vi "Q.Send Function Command and wait on Ret Data.vi"(5 "Timeout(ms)":i32=100, 7 "Q Name":string, 8 "error in":errorcluster, 9 "Data1":variant, 10 "Cmd":string, 11 "Q In":refnum<queue>) -> (0 "error out":errorcluster, 2 "Ret":variant)   [LabVIEW 2024, in "EQMF.lvlib" / "Queue Utils.lvlib"]
uses:
  Queue Utils.lvlib
  Q.Element.ctl
  Q.Msg Return Info.ctl
  Q.Msg Return Data Container.ctl
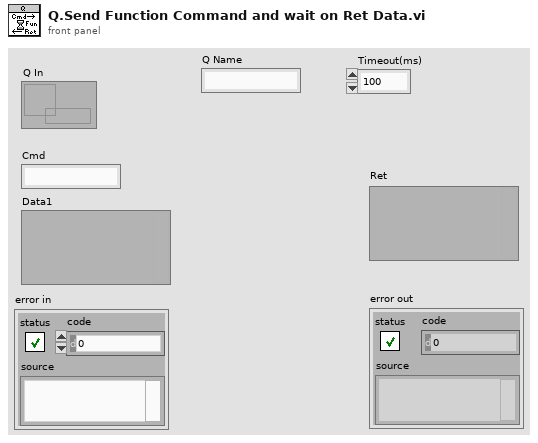
[diagram p1: front panel]
types:
  T1 = typedef "EQMF.lvlib/Queue Utils.lvlib/Q.Msg Return Info.ctl" = cluster{"Ret Q":refnum<queue>, "Ret Msg":T2, "SeqNum":i32}
  T2 = typedef "EQMF.lvlib/Queue Utils.lvlib/Q.Element.ctl" = cluster{"Cmd":string, "Sub":string, "Data1":variant, "Data2":variant}
  T3 = typedef "EQMF.lvlib/Queue Utils.lvlib/Q.Msg Return Data Container.ctl" = cluster{"SeqNum":i32, "Data":variant, "Error":errorcluster}
  T4 = cluster{"Q Cmd":refnum<queue>, "Q Ret":refnum<queue>, "Q Name":string, "Cmd ":string, "State":string, "Ret":variant}
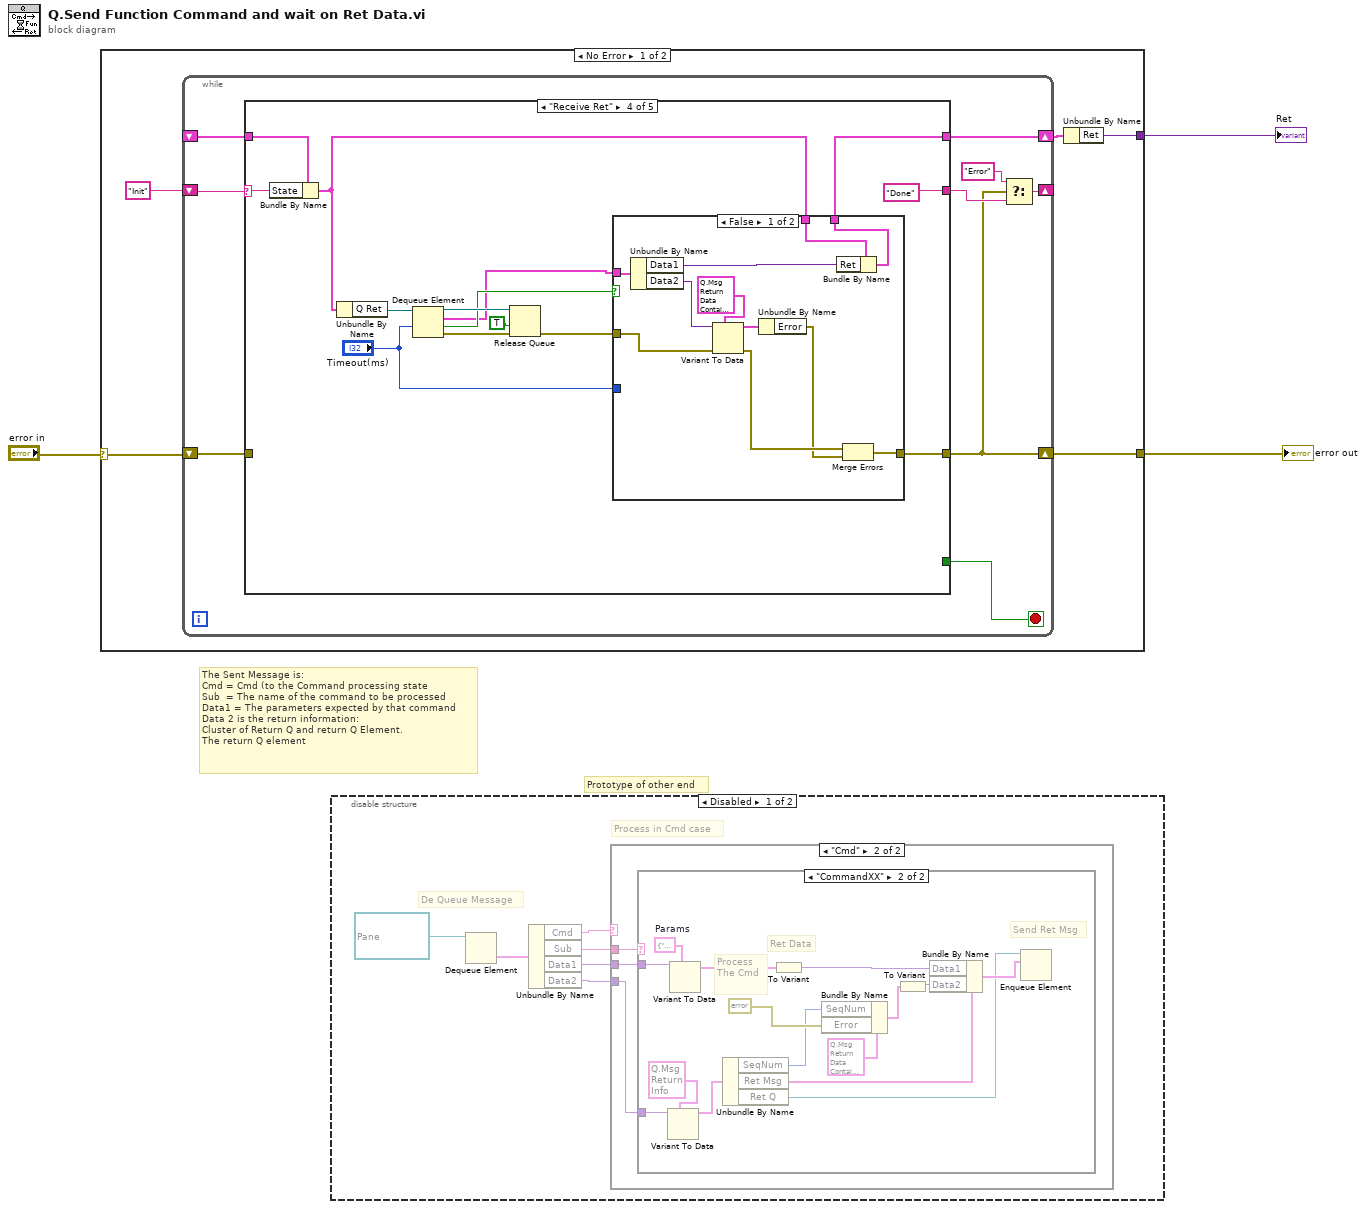
[diagram p0: block diagram]
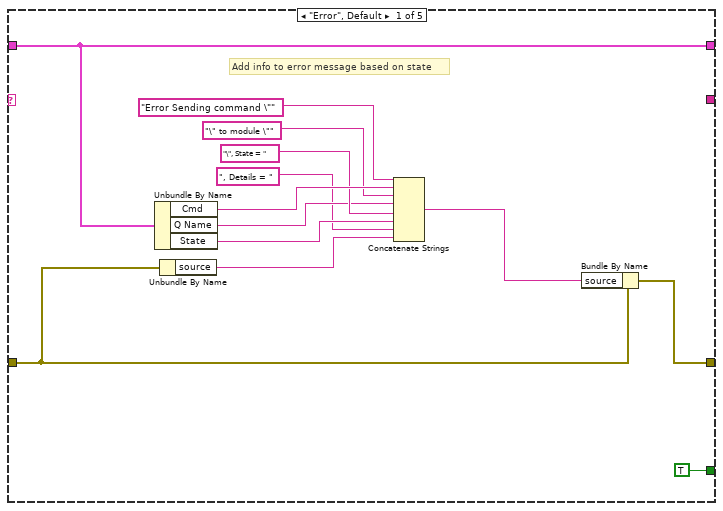
[diagram p2: hidden frame]
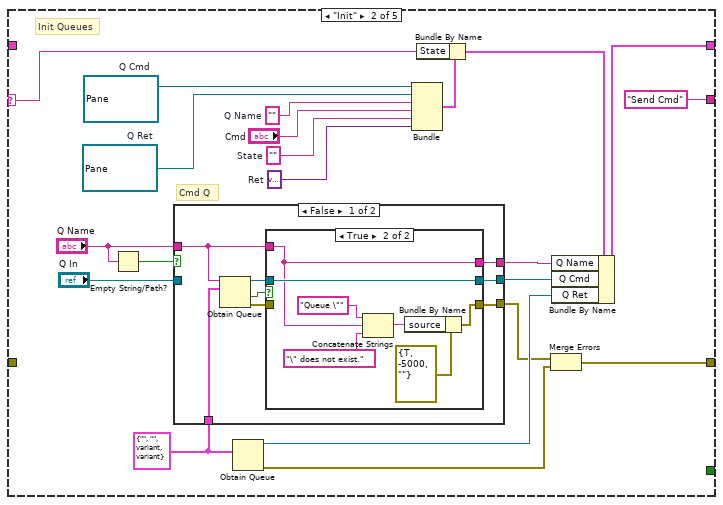
[diagram p3: hidden frame]
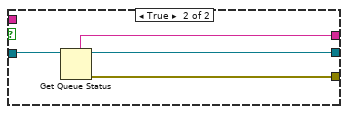
[diagram p5: hidden frame]
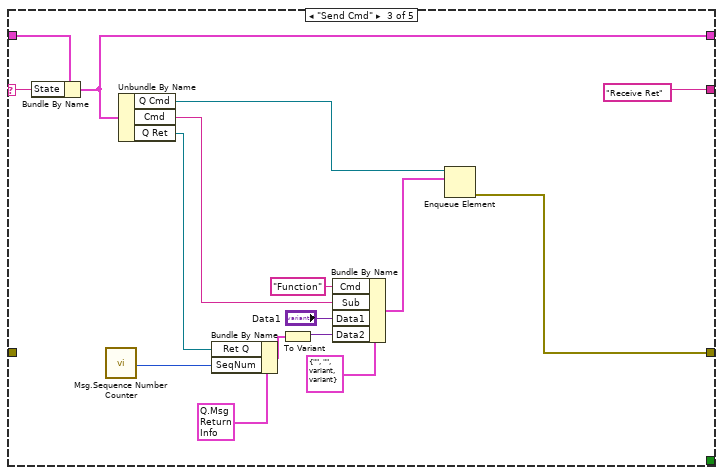
[diagram p6: hidden frame]
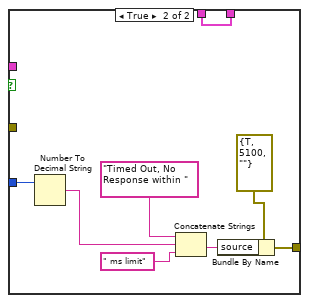
[diagram p7: hidden frame]
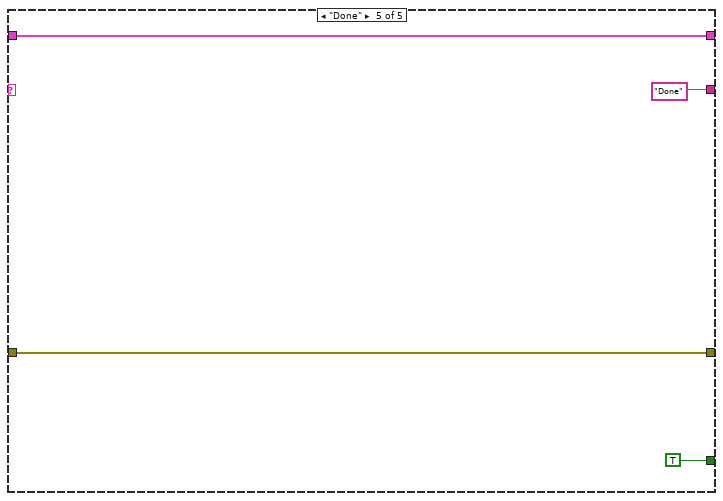
[diagram p8: hidden frame]
diagram:
  # "Prototype of other end"
  # "The Sent Message is:\nCmd = Cmd (to the Command processing state\nSub  = The name of the command to be processed\nData1 = The parameters expected by that command\nData 2 is the return information:\nCluster of Return Q and return Q Element.\nThe return Q element"
  n1 = case shown="No Error" "error in" {
    selector: "error in" -> [w7 w127]
    tunnel: [w6 w127] -> w2
    tunnel: [w4 _] -> w1
    frame No Error {
      n2 = while {
        shift-right: [w15] -> w5
        shift-left: _ -> [w17]
        shift-right: [w12] -> _
        shift-left: "Init" -> [w16]
        shift-right: [w10] -> w6
        shift-left: w7 -> [w9]
        stop <- w11 stop-if-true
        n3 = case shown="\"Receive Ret\"" w16 {
          selector: w16 -> [_ w33 w79 w103 _]
          tunnel: w17 -> [w29 _ w78 w102 w124]
          tunnel: [w29 w32 w77 w90 w124] -> w15
          tunnel: [_ "Send Cmd" "Receive Ret" "Done" "Done"] -> w13
          tunnel: [w28 w38 w75 w95 w123] -> w10
          tunnel: [TRUE _ _ _ TRUE] -> w11
          tunnel: w9 -> [w27 _ _ _ w123]
          frame "Error", Default {
            # "Add info to error message based on state"
            n4 = Unbundle By Name(w29) -> ("Cmd"=w25:string, "Q Name"=w22:string, "State"=w21:string)
            n5 = Unbundle By Name(w27) -> ("source"=w19:string)
            n6 = Concatenate Strings("Error Sending command \"", w25, "\" to module \"", w22, "\", State = ", w21, ", Details = ", w19) -> (w18:string)
            n7 = Bundle By Name(cluster=w27, "source"=w18) -> (w28:errorcluster)
          }
          frame "Init" {
            w31 = variant  # Ret
            w37 = ""  # State
            w43 = ""  # Q Name
            w46 = refnum<queue> refnum  # Q Ret
            w47 = refnum<queue> refnum  # Q Cmd
            w48 = T2 {"Cmd"="", "Sub"="", "Data1"=variant, "Data2"=variant}
            # "Cmd Q"
            # "Init Queues"
            n8 = Empty String/Path?(string/path="Q Name") -> (empty?=w51:bool)
            n9 = case shown="False" w51 {
              tunnel: "Q Name" -> [w53 _]
              tunnel: "Q In" -> [_ w72]
              tunnel: w48 -> [w59 _]
              tunnel: [w55 w73] -> w45
              tunnel: [w52 w71] -> w42
              tunnel: [w54 w70] -> w40
              frame False {
                n10 = Obtain Queue(name (unnamed)=w53, element data type=w59) -> (queue out=w57:refnum<queue>, created new?=w58:bool, error out=w56:errorcluster)  [unwired: 3 in]
                n11 = case shown="True" w58 {
                  tunnel: w57 -> [w62 w64]
                  tunnel: w56 -> [w61 _]
                  tunnel: [w62 w64] -> w55
                  tunnel: [w61 w65] -> w54
                  tunnel: w53 -> [w60 w63]
                  tunnel: [w60 w63] -> w52
                  frame False {
                  }
                  frame True {
                    n12 = Concatenate Strings("Queue \"", w63, "\" does not exist.") -> (w66:string)
                    n13 = Bundle By Name(cluster=errorcluster {"status"=TRUE, "code"=-5000, "source"=""} ("error constant"), "source"=w66) -> (w65:errorcluster)
                  }
                }
              }
              frame True {
                n14 = Get Queue Status(queue=w72) -> (queue out=w73:refnum<queue>, queue name=w71:string, error out=w70:errorcluster)  [unwired: 2 in, 5 out]
              }
            }
            n15 = Obtain Queue(element data type=w48) -> (queue out=w44:refnum<queue>, error out=w39:errorcluster)  [unwired: 4 in, 1 out]
            n16 = Bundle("Q Cmd"=w47, "Q Ret"=w46, "Q Name"=w43, "Cmd"="Cmd", "State"=w37, "Ret"=w31) -> (w35:T4)  [unwired: 1 in]
            n17 = Bundle By Name(cluster=w35, "State"=w33) -> (w34:T4)
            n18 = Merge Errors(w40, w39) -> (w38:errorcluster)
            n19 = Bundle By Name(cluster=w34, "Q Name"=w42, "Q Cmd"=w45, "Q Ret"=w44) -> (w32:T4)
          }
          frame "Send Cmd" {
            n20 = Bundle By Name(cluster=w78, "State"=w79) -> (w77:T4)
            n21 = call "Msg.Sequence Number Counter.vi"() -> ("SeqNum"=w74:i32)  [unwired: 1 in]
            n22 = Unbundle By Name(w77) -> ("Q Cmd"=w86:refnum<queue>, "Cmd"=w84:string, "Q Ret"=w81:refnum<queue>)
            n23 = Bundle By Name(cluster=T1 {"Ret Q"=refnum, "Ret Msg"={"Cmd"="", "Sub"="", "Data1"=variant, "Data2"=variant}, "SeqNum"=0} ("Cmd Ret Req Data"), "Ret Q"=w81, "SeqNum"=w74) -> (w80:T1)
            n24 = To Variant(anything=w80) -> (Variant=w85:variant)
            n25 = Bundle By Name(cluster=T2 {"Cmd"="", "Sub"="", "Data1"=variant, "Data2"=variant}, "Cmd"="Function", "Sub"=w84, "Data1"="Data1", "Data2"=w85) -> (w83:T2)
            n26 = Enqueue Element(queue=w86, element=w83) -> (error out=w75:errorcluster)  [unwired: 2 in, 2 out]
          }
          frame "Receive Ret" {
            n27 = Bundle By Name(cluster=w102, "State"=w103) -> (w91:T4)
            n28 = Unbundle By Name(w91) -> ("Q Ret"=w101:refnum<queue>)
            n29 = Dequeue Element(queue=w101, timeout in ms (-1)="Timeout(ms)") -> (queue out=w100:refnum<queue>, element=w92:T2, timed out?=w96:bool, error out=w99:errorcluster)  [unwired: 1 in]
            n30 = Release Queue(queue=w100, force destroy? (F)=TRUE, error in (no error)=w99) -> (error out=w97:errorcluster)  [unwired: 2 out]
            n31 = case shown="False" w96 {
              tunnel: w97 -> [w109 _]
              tunnel: [w106 w121] -> w95
              tunnel: "Timeout(ms)" -> [_ w116]
              tunnel: w92 -> [w110 _]
              tunnel: w91 -> [w108 w115]
              tunnel: [w107 w115] -> w90
              frame False {
                n32 = Unbundle By Name(w110) -> ("Data1"=w114:variant, "Data2"=w113:variant)
                n33 = Variant To Data(error in=w109, type=T3 {"SeqNum"=0, "Data"=variant, "Error"={"status"=FALSE, "code"=0, "source"=""}} ("Ret"), Variant=w113) -> (data=w111:T3, error out=w105:errorcluster)
                n34 = Unbundle By Name(w111) -> ("Error"=w104:errorcluster)
                n35 = Bundle By Name(cluster=w108, "Ret"=w114) -> (w107:T4)
                n36 = Merge Errors(w105, w104) -> (w106:errorcluster)
              }
              frame True {
                n37 = Number To Decimal String(number=w116) -> (decimal integer string=w118:string)  [unwired: 1 in]
                n38 = Concatenate Strings("Timed Out, No Response within ", w118, " ms limit") -> (w120:string)
                n39 = Bundle By Name(cluster=errorcluster {"status"=TRUE, "code"=5100, "source"=""} ("error constant"), "source"=w120) -> (w121:errorcluster)
              }
            }
          }
          frame "Done" {
          }
        }
        n40 = Select(t="Error", s=w10, f=w13) -> (s? t:f=w12:string)
      }
      n41 = Unbundle By Name(w5) -> ("Ret"=w4:variant)
    }
    frame Error {
    }
  }
  "error out" <- w2
  "Ret" <- w1
  n42 = disable-structure shown="Disabled" {
    frame Disabled {
      # "Process in Cmd case"
      # "De Queue Message"
      n43 = Dequeue Element(queue=refnum<queue> refnum ("Q Cmd")) -> (element=w132:T2)  [unwired: 2 in, 3 out]
      n44 = Unbundle By Name(w132) -> ("Cmd"=w131:string, "Sub"=w130:string, "Data1"=w129:variant, "Data2"=w128:variant)
      n45 = case shown="\"Cmd\"" w131 {
        tunnel: w130 -> [_ w136]
        tunnel: w129 -> [_ w135]
        tunnel: w128 -> [_ w134]
        frame "False", Default {
        }
        frame "Cmd" {
          n46 = case shown="\"CommandXX\"" w136 {
            tunnel: w135 -> [_ w151]
            tunnel: w134 -> [_ w149]
            frame "False", Default {
            }
            frame "CommandXX" {
              w150 = cluster{string, string} {"", ""}  # Params
              # "Send Ret Msg"
              # "Ret Data"
              # "Process \nThe Cmd"
              n47 = Variant To Data(type=T1 {"Ret Q"=refnum, "Ret Msg"={"Cmd"="", "Sub"="", "Data1"=variant, "Data2"=variant}, "SeqNum"=0} ("Cmd Ret Req Data"), Variant=w149) -> (data=w147:T1)  [unwired: 1 in, 1 out]
              n48 = Variant To Data(type=w150, Variant=w151) -> (data=w144:cluster{string, string})  [unwired: 1 in, 1 out]
              n49 = Unbundle By Name(w147) -> ("SeqNum"=w139:i32, "Ret Msg"=w146:T2, "Ret Q"=w142:refnum<queue>)
              n50 = To Variant(anything=w144) -> (Variant=w145:variant)
              n51 = Bundle By Name(cluster=T3 {"SeqNum"=0, "Data"=variant, "Error"={"status"=FALSE, "code"=0, "source"=""}} ("Ret"), "SeqNum"=w139, "Error"=errorcluster {"status"=FALSE, "code"=0, "source"=""} ("error constant")) -> (w137:T3)
              n52 = To Variant(anything=w137) -> (Variant=w138:variant)
              n53 = Bundle By Name(cluster=w146, "Data1"=w145, "Data2"=w138) -> (w143:T2)
              n54 = Enqueue Element(queue=w142, element=w143) -> ()  [unwired: 2 in, 3 out]
            }
          }
        }
      }
    }
    frame Enabled {
    }
  }
